vi "Arm raise.vi"(8 "Power":i8=-30, 10 "Rotation":i32=70, 11 "EV3 in":T1) -> (3 "EV3 out":T1)   [LabVIEW 2016]
uses:
  <vilib>/NXT/Subs/LVHSConnector.ctl
  <vilib>/NXT/LegoClasses/BrickReference/BrickReference.lvclass
  <vilib>/NXT/Block Support/NXT_OutputPort.ctl
  <vilib>/NXT/NXTIO Xnodes/NXTIONodeSubVIs/LEGOResetMotors.vi
  <vilib>/NXT/NXTIO Xnodes/NXTIONodeSubVIs/NXTMotorRunDistance.vi
  <vilib>/NXT/Dual Mode Library/Waits/Wait_Num.vi
  <vilib>/NXT/NXTIO Xnodes/NXTIOXNode/NXTIO.xnode
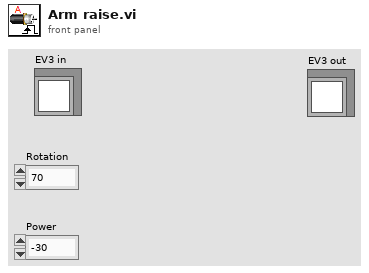
[diagram p1: front panel]
types:
  T1 = typedef "LVHSConnector.ctl" = refnum<class "BrickReference.lvclass">
  T2 = typedef "NXT_OutputPort.ctl" = u8
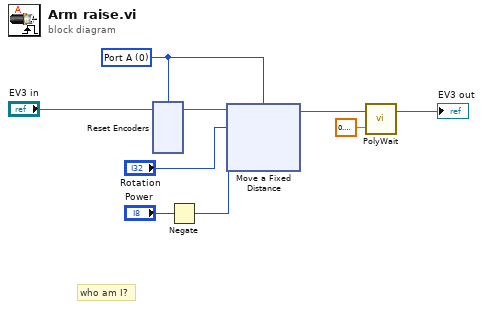
[diagram p0: block diagram]
diagram:
  w7 = T2 0 items=["Port A", "Port B", "Port C", "Port D"] ("Motors")
  # "who am I?"
  n1 = xnode "Reset Encoders"("Motors"=w7, "NXT/EV3"="EV3 in") -> ("NXT/EV3"=w6:T1)
  n2 = Negate(x="Power") -> (-x=w3:i8)
  n3 = xnode "Move a Fixed Distance"("Speed 1"=w3, "Distance 1"="Rotation", "Motors"=w7, "NXT/EV3"=w6) -> ("NXT/EV3"=w8:T1)
  n4 = call-poly <vilib>:"PolyWait.vi"("Time (1 sec)"=sgl 0.2, "NXT/EV3"=w8) -> ("NXT/EV3"=→"EV3 out":T1)  [unwired: 2 in]
